vi "Read_fifo_cmd_backup.vi"(8 "error in (no error)":errorcluster, 10 "FIFO_pkt_size":u32=4096, 11 "VISA Refnum in":refnum<visa-resource-name>) -> (0 "error out":errorcluster, 1 "Data_out":u8[](array[numeric]), 3 "VISA Refnum out":refnum<visa-resource-name>)   [LabVIEW 2019]
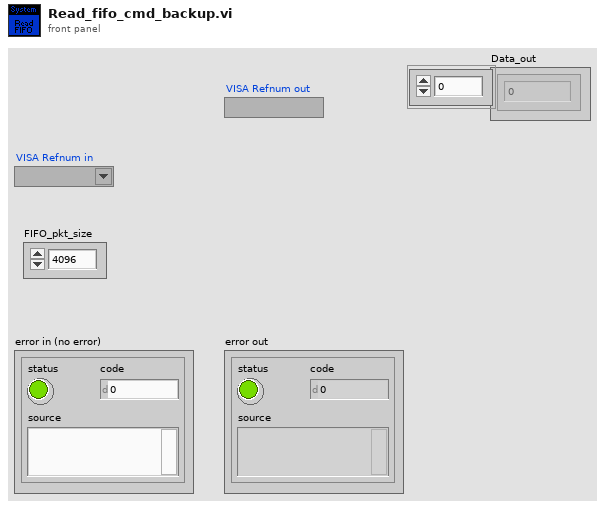
[diagram p1: front panel]
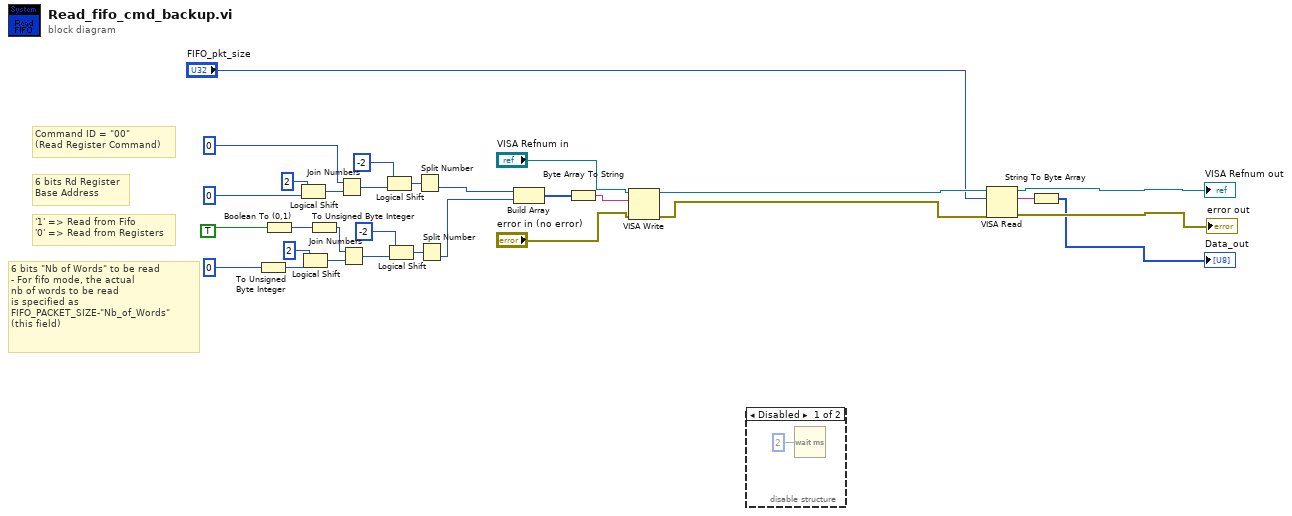
[diagram p0: block diagram]
diagram:
  # "'1' => Read from Fifo\n'0' => Read from Registers"
  # "6 bits \"Nb of Words\" to be read\n- For fifo mode, the actual \nnb of words to be read \nis specified as \nFIFO_PACKET_SIZE-\"Nb_of_Words\" \n(this field)"
  # "6 bits Rd Register \nBase Address"
  # "Command ID = \"00\" \n(Read Register Command)"
  n1 = To Unsigned Byte Integer(number=u8 0 ("t")) -> (unsigned 8bit integer=w9:u8)
  n2 = Boolean To (0,1)(Boolean=TRUE ("Fifo-mode En")) -> (0, 1=w13:i16)
  n3 = Logical Shift(y=i16 2, x=u8 0 ("RdReg Addr")) -> (x << y=w24:u8)
  n4 = Logical Shift(y=i16 2, x=w9) -> (x << y=w17:u8)
  n5 = To Unsigned Byte Integer(number=w13) -> (unsigned 8bit integer=w12:u8)
  n6 = Join Numbers(hi=u8 0, lo=w24) -> ((hi.lo)=w25:u16)
  n7 = Join Numbers(hi=w12, lo=w17) -> ((hi.lo)=w16:u16)
  n8 = Logical Shift(y=i16 -2, x=w25) -> (x << y=w21:u16)
  n9 = Logical Shift(y=i16 -2, x=w16) -> (x << y=w19:u16)
  n10 = Split Number(x=w21) -> (lo(x)=w20:u8)  [unwired: 1 out]
  n11 = Split Number(x=w19) -> (lo(x)=w14:u8)  [unwired: 1 out]
  n12 = Build Array(w20, w14) -> (w10:u8[])
  n13 = Byte Array To String(unsigned byte array=w10) -> (string=w11:string)
  n14 = VISA Write(VISA resource name="VISA Refnum in", write buffer=w11, error in (no error)="error in (no error)") -> (VISA resource name out=w4:refnum<visa-resource-name>, error out=w5:errorcluster)  [unwired: 1 out]
  n15 = disable-structure shown="Disabled" {
    frame Disabled {
      n16 = Wait (ms)(milliseconds to wait=u32 2) -> ()  [unwired: 1 out]
    }
    frame Enabled {
    }
  }
  n17 = VISA Read(VISA resource name=w4, byte count="FIFO_pkt_size", error in (no error)=w5) -> (VISA resource name out=→"VISA Refnum out":refnum<visa-resource-name>, read buffer=w2:string, error out=→"error out":errorcluster)  [unwired: 1 out]
  n18 = String To Byte Array(string=w2) -> (unsigned byte array=→"Data_out":u8[])
